vi "ppanel_generate_user_events.vi"(8 "error in (no error)":errorcluster, 11 "picoharp_panel in":refnum<class "picoharp_panel.lvclass">) -> (0 "error out":errorcluster, 2 "events":T1, 3 "hydraharp_panel out":refnum<class "picoharp_panel.lvclass">)   [LabVIEW 2015, in "picoharp_panel.lvclass"]
uses:
  picoharp_panel.lvclass
  Hydraharp/hydraharp_panel/hpanel_user_events.ctl
  Hydraharp/hydraharp_panel/hpanel_messages_to_panel_from_actor_loop.ctl
  ppanel_user_events.ctl
  picoharp_panel.lvclass/picoharp_panel.ctl
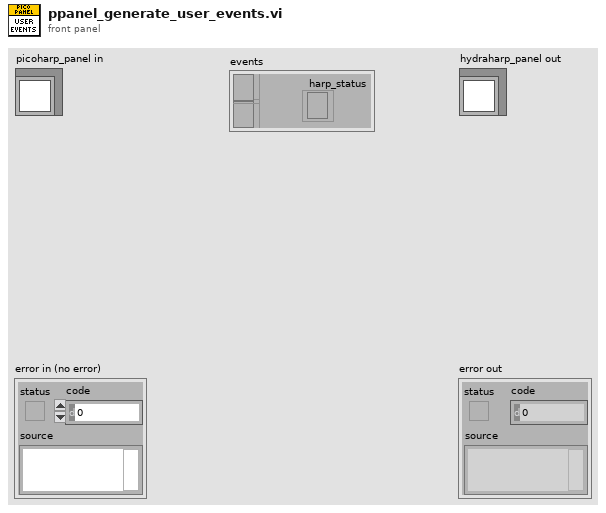
[diagram p1: front panel]
types:
  T1 = typedef "hpanel_user_events.ctl" = cluster{"message_panel":refnum<event-registration>, "stop_fifo_stream":refnum<event-registration>, "harp_status":refnum<event-registration>}
  T2 = typedef "ppanel_user_events.ctl" = cluster{"message_panel":refnum<event-registration>, "stop_fifo_stream":refnum<event-registration>, "update_picoharp_status":refnum<event-registration>}
  T3 = typedef "hpanel_messages_to_panel_from_actor_loop.ctl" = enum16{"reenable_tasks"}
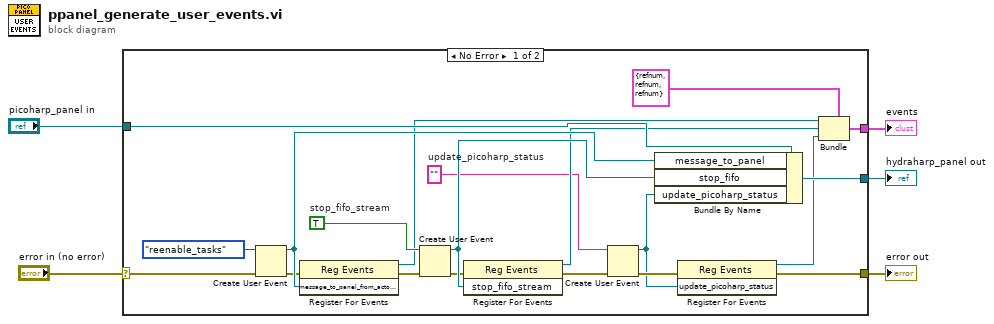
[diagram p0: block diagram]
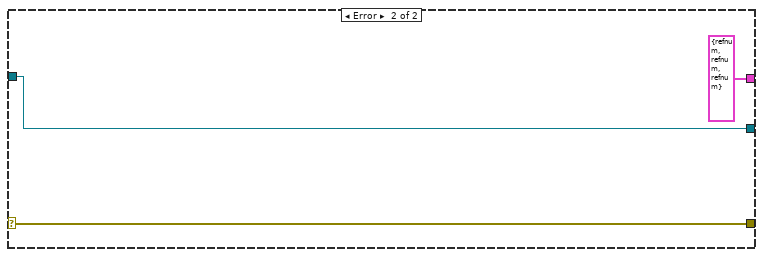
[diagram p2: hidden frame]
diagram:
  n1 = case shown="No Error" "error in (no error)" {
    selector: "error in (no error)" -> [w24 w28]
    tunnel: [w9 w28] -> w4
    tunnel: [w21 w27] -> w2
    tunnel: "picoharp_panel in" -> [w23 w27]
    tunnel: [w16 T1 {"message_panel"=refnum, "stop_fifo_stream"=refnum, "harp_status"=refnum} ("output cluster")] -> w1
    frame No Error {
      w11 = ""  # update_picoharp_status
      w20 = TRUE  # stop_fifo_stream
      n2 = Create User Event(user event datatype=hpanel_messages_to_panel_from_actor_loop."reenable_tasks" ("message_to_panel_from_actor_loop"), error in=w24) -> (user event=w22:refnum<user-event>, error out=w15:errorcluster)
      n3 = register-events(error in=w15, w22) -> (reference out=w17:refnum<event-registration>, error out=w14:errorcluster)  [unwired: 1 in]
      n4 = Create User Event(user event datatype=w20, error in=w14) -> (user event=w19:refnum<user-event>, error out=w13:errorcluster)
      n5 = register-events(error in=w13, w19) -> (reference out=w18:refnum<event-registration>, error out=w12:errorcluster)  [unwired: 1 in]
      n6 = Create User Event(user event datatype=w11, error in=w12) -> (user event=w8:refnum<user-event>, error out=w10:errorcluster)
      n7 = Bundle By Name(cluster=w23, "message_to_panel"=w22, "stop_fifo"=w19, "update_picoharp_status"=w8) -> (w21:refnum<class "picoharp_panel.lvclass">)
      n8 = register-events(error in=w10, w8) -> (reference out=w7:refnum<event-registration>, error out=w9:errorcluster)  [unwired: 1 in]
      n9 = Bundle(cluster=T2 {"message_panel"=refnum, "stop_fifo_stream"=refnum, "update_picoharp_status"=refnum} ("output cluster"), "message_panel"=w17, "stop_fifo_stream"=w18, "update_picoharp_status"=w7) -> (w16:T2)
    }
    frame Error {
    }
  }
  "error out" <- w4
  "hydraharp_panel out" <- w2
  "events" <- w1
